vi "drawbg.vi"(10 "size":i32, 11 "2D Picture":picture) -> (2 "Cluster":T1, 3 "new picture":picture)   [LabVIEW 2025]
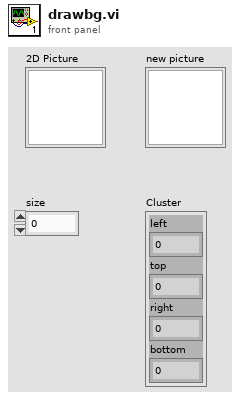
[diagram p1: front panel]
types:
  T1 = cluster{"left":i16, "top":i16, "right":i16, "bottom":i16}
  T2 = cluster{"Width":i16, "Style":enum32{"Solid", "Dash", "Dot", "DashDot", "DashDotDot"}}
  T3 = cluster{"Width":u16, "Style":enum32{"Solid", "Dash", "Dot", "DashDot", "DashDotDot"}}
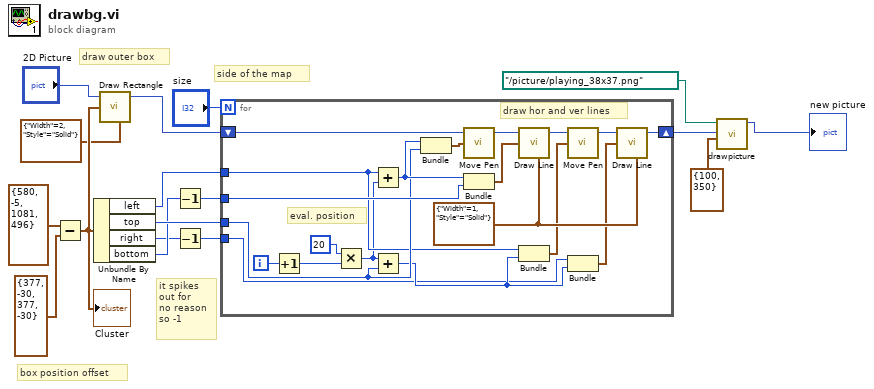
[diagram p0: block diagram]
diagram:
  # "it spikes\nout for \nno reason\nso -1"
  # "box position offset"
  # "side of the map"
  # "draw outer box"
  n1 = Subtract(x=T1 {"left"=580, "top"=-5, "right"=1081, "bottom"=496} ("rect"), y=T1 {"left"=377, "top"=-30, "right"=377, "bottom"=-30}) -> (x-y=w17:T1)
  "Cluster" <- w17
  n2 = Unbundle By Name(w17) -> ("left"=w14:i16, "top"=w13:i16, "right"=w9:i16, "bottom"=w11:i16)
  n3 = call <vilib>:"Draw Rectangle.vi"("picture"="2D Picture", "rect"=w17, "pen"=T2 {"Width"=2, "Style"=enum."Solid"}) -> ("new picture"=w8:picture)  [unwired: 6 in]
  n4 = Decrement(x=w11) -> (x-1=w12:i16)
  n5 = Decrement(x=w9) -> (x-1=w10:i16)
  n6 = for {
    N: "size" -> [_]
    shift-right: [w37] -> w4
    shift-left: w8 -> [w34]
    tunnel: w14 -> [w25]
    tunnel: w13 -> [w26]
    tunnel: w10 -> [w22]
    tunnel: w12 -> [w29]
    i -> [w19]
    w36 = T3 {"Width"=1, "Style"=enum."Solid"} ("pen")
    # "eval. position"
    # "draw hor and ver lines"
    n7 = Increment(x=w19) -> (x+1=w18:i32)
    n8 = Multiply(x=20, y=w18) -> (x*y=w20:i32)
    n9 = Add(x=w25, y=w20) -> (x+y=w28:i32)
    n10 = Add(x=w20, y=w26) -> (x+y=w23:i32)
    n11 = Bundle(w28, "top"=w26) -> (w30:cluster{i32, "top":i16})  [unwired: 1 in]
    n12 = call <vilib>:"Move Pen.vi"("new position"=w30, "picture"=w34) -> ("new picture"=w33:picture)  [unwired: 3 in]
    n13 = Bundle(w28, w29) -> (w27:cluster{i32, i16})  [unwired: 1 in]
    n14 = call <vilib>:"Draw Line.vi"("picture"=w33, "end point"=w27, "pen"=w36) -> ("new picture"=w35:picture)  [unwired: 6 in]
    n15 = Bundle("left"=w25, w23) -> (w24:cluster{"left":i16, i32})  [unwired: 1 in]
    n16 = call <vilib>:"Move Pen.vi"("new position"=w24, "picture"=w35) -> ("new picture"=w32:picture)  [unwired: 3 in]
    n17 = Bundle(w22, w23) -> (w21:cluster{i16, i32})  [unwired: 1 in]
    n18 = call <vilib>:"Draw Line.vi"("picture"=w32, "end point"=w21, "pen"=w36) -> ("new picture"=w37:picture)  [unwired: 6 in]
  }
  n19 = call "drawpicture.vi"("y"=cluster{"left":i16, "top":i16} {"left"=100, "top"=350}, "2D Picture"=w4, "name or relative path"=path "../picture/playing_38x37.png") -> ("new picture"=→"new picture":picture)  [unwired: 8 in]
